vi "ROI_saving.vi"() -> ()   [LabVIEW 2025]
uses:
  <vilib>/vision/NI_Vision_Development_Module.lvlib
panel:
  in  "Image Name":string="untitled3.jpg"
  out "Image 2":T1(plugin-control)
  out "error out":errorcluster
  in  "ROI Path":path
  in  "stop":bool
  out "Global Rectangle":i32[](array[numeric])
  out "Image":T1(plugin-control)
  in  "File Path":path
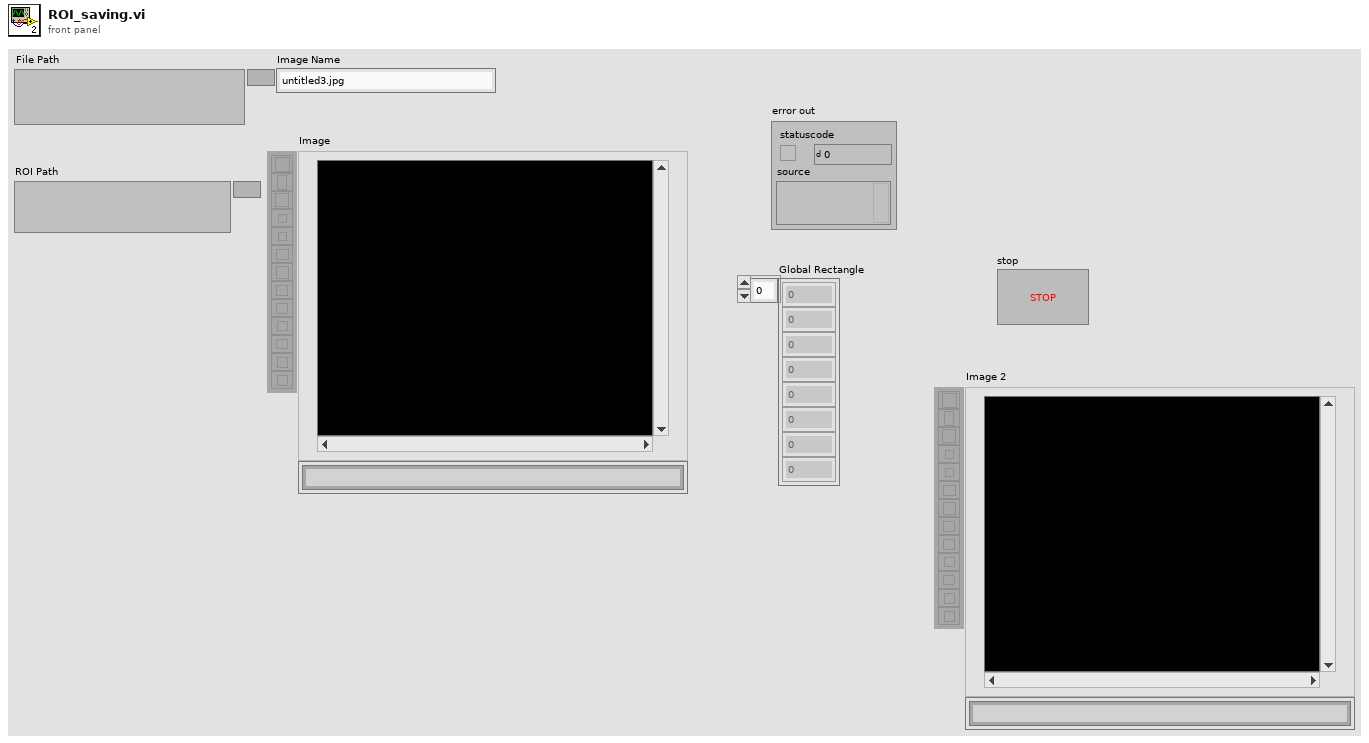
[diagram p1: front panel]
types:
  T1 = typedef "IMAQ Image.ctl" = refnum<image>
  T2 = typedef "Image Type" = u32
  T3 = cluster{"Global Rectangle":i32[], "Contours":cluster{"Contour Type":u32, "ROI Type":u32, "Points":i32[]}[]}
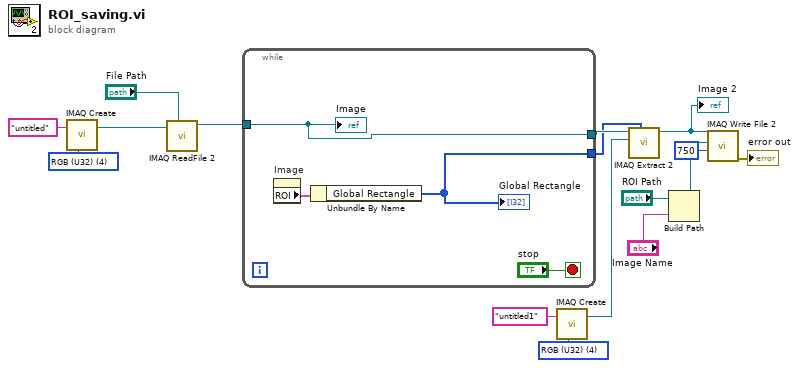
[diagram p0: block diagram]
diagram:
  w10 = T2 4 items=["Grayscale (U8)", "Grayscale (I16)", "Grayscale (SGL)", "Complex (CSG)", "RGB (U32)", "HSL (U32)", "RGB (U64)", "Grayscale (U16)"] ("Image Type")
  w15 = T2 4 items=["Grayscale (U8)", "Grayscale (I16)", "Grayscale (SGL)", "Complex (CSG)", "RGB (U32)", "HSL (U32)", "RGB (U64)", "Grayscale (U16)"] ("Image Type")
  n1 = call "IMAQ Create"("Image Name"="untitled", "Image Type"=w15) -> ("New Image"=w14:T1)  [unwired: 3 in, 1 out]
  n2 = call "IMAQ ReadFile 2"("File Path"="File Path", "Image"=w14) -> ("Image Out"=w12:T1)  [unwired: 5 in, 4 out]
  n3 = while {
    tunnel: w12 -> [w18]
    tunnel: [w18] -> w11
    tunnel: [w17] -> w7
    stop <- "stop" stop-if-true
    n4 = property on="Image" class="ImageControl"() -> ("ROI"=w20:T3)  [unwired: 2 in, 2 out]
    n5 = Unbundle By Name(w20) -> ("Global Rectangle"=w17:i32[])
    "Global Rectangle" <- w17
    "Image" <- w18
  }
  n6 = call "IMAQ Create"("Image Name"="untitled1", "Image Type"=w10) -> ("New Image"=w8:T1)  [unwired: 3 in, 1 out]
  n7 = call "IMAQ Extract 2"("Optional Rectangle"=w7, "Image Dst"=w8, "Image Src"=w11) -> ("Image Dst Out"=w1:T1)  [unwired: 7 in, 1 out]
  "Image 2" <- w1
  n8 = Build Path(base path="ROI Path", name or relative path="Image Name") -> (appended path=w3:path)
  n9 = call-poly "IMAQ Write File 2"("Image Quality"=u32 750, "File Path"=w3, "Image"=w1) -> ("error out"=→"error out":errorcluster)  [unwired: 7 in, 1 out]
